vi "VerifyArgumentsCore.vi"(8 "error in (no error)":errorcluster, 11 "ExecuteAllBuildSpecsWithVersion in":refnum<class "ExecuteAllBuildSpecsWithVersion.lvclass">) -> (0 "error out":errorcluster, 3 "ExecuteAllBuildSpecsWithVersion out":refnum<class "ExecuteAllBuildSpecsWithVersion.lvclass">)   [LabVIEW 2015, in "ExecuteAllBuildSpecsWithVersion.lvclass"]
doc: "VI to be overridden by child classes to validate operation-specific arguments."
uses:
  ExecuteAllBuildSpecsWithVersion.lvclass
  ExecuteAllBuildSpecsWithVersion.lvclass/ExecuteAllBuildSpecsWithVersion.ctl
  <nishared>/LabVIEW CLI/Operations/Utilities/OperationErrorType.ctl
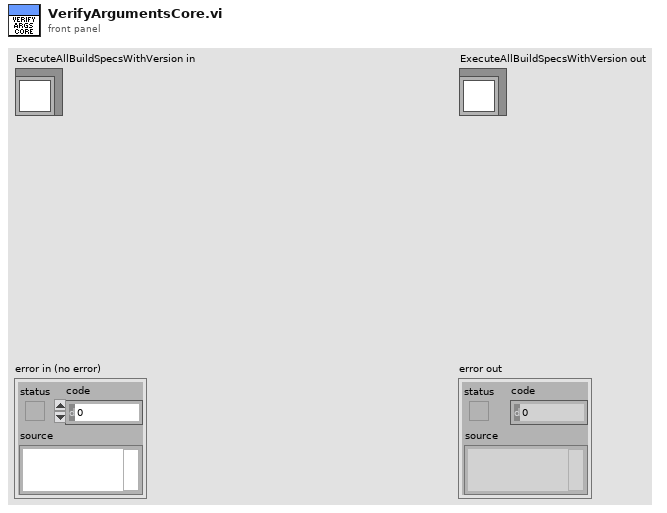
[diagram p1: front panel]
types:
  T1 = typedef "OperationErrorType.ctl" = enum16{"RequiredArgumentMissing", "UnknownArguments", "LoggerSetMultipleTimes", "OperationBrokenError"}
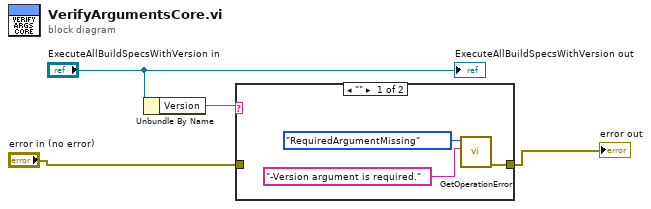
[diagram p0: block diagram]
diagram:
  n1 = Unbundle By Name("ExecuteAllBuildSpecsWithVersion in") -> ("Version"=w2:string)
  n2 = case shown="\"\"" w2 {
    tunnel: [w7 w8] -> w3
    tunnel: "error in (no error)" -> [_ w8]
    frame "" {
      n3 = call <nishared>:"GetOperationError.vi"("Additional Information"="-Version argument is required.", "Operation Error Type"=OperationErrorType."RequiredArgumentMissing") -> ("error out"=w7:errorcluster)  [unwired: 9 in]
    }
    frame Default {
    }
  }
  "error out" <- w3
  "ExecuteAllBuildSpecsWithVersion out" <- "ExecuteAllBuildSpecsWithVersion in"
